vi "Set Combobox Items.vi"(6 "Combo Box Ref":refnum<vi>, 8 "error in (no error)":errorcluster, 9 "Run Mode?":bool, 10 "Indicator?":bool, 11 "Static Path Selector in":refnum<class "MGI Static Path Selector.lvclass">) -> (0 "error out":errorcluster, 2 "Strings And Values []":T1, 3 "Static Path Selector out":refnum<class "MGI Static Path Selector.lvclass">)   [LabVIEW 2020, in "MGI Static Path Selector.lvclass"]
doc: "Sets the Combobox strings to appropriate values for the specified state of the XControl.\n\nAuthored by Shawn Walpole\nsupport@mooregoodideas.com\nwww.mooregoodideas.com\n\nCopyright (c) 2013, Moore Good Ideas, Inc.\n\nAll rights reserved.\n\nRedistribution and use in source and binary forms, with or without modification, are permitted provided that the following conditions are met:\n\n * Redistributions of source code must retain the above copyright notice, this list of conditions and the following disclaimer.\n * Redistributions in binary form must reproduce the above copyright notice, this list of conditions and the following disclaimer in the documentation and/or other materials provided with the distribution.\n * Neither the name of Moore Good Ideas, Inc. nor the names of its contributors may be used to endorse or promote products derived from this software without specific prior written permission.\n\nTHIS SOFTWARE IS PROVIDED BY THE COPYRIGHT HOLDERS AND CONTRIBUTORS \"AS IS\" AND ANY EXPRESS OR IMPLIED WARRANTIES, INCLUDING, BUT NOT LIMITED TO, THE IMPLIED WARRANTIES OF MERCHANTABILITY AND FITNESS FOR A PARTICULAR PURPOSE ARE DISCLAIMED. IN NO EVENT SHALL THE COPYRIGHT OWNER OR CONTRIBUTORS BE LIABLE FOR ANY DIRECT, INDIRECT, INCIDENTAL, SPECIAL, EXEMPLARY, OR CONSEQUENTIAL DAMAGES (INCLUDING, BUT NOT LIMITED TO, PROCUREMENT OF SUBSTITUTE GOODS OR SERVICES; LOSS OF USE, DATA, OR PROFITS; OR BUSINESS INTERRUPTION) HOWEVER CAUSED AND ON ANY THEORY OF LIABILITY, WHETHER IN CONTRACT, STRICT LIABILITY, OR TORT (INCLUDING NEGLIGENCE OR OTHERWISE) ARISING IN ANY WAY OUT OF THE USE OF THIS SOFTWARE, EVEN IF ADVISED OF THE POSSIBILITY OF SUCH DAMAGE."
uses:
  <userlib>/_MGI/User Interface/Path Selector XControl/Class Hierarchy/Static File Selector/MGI Static Path Selector.lvclass
  <vilib>/Utility/miscctls.llb/LVComboBoxStrsAndValuesArrayTypeDef.ctl
  <userlib>/_MGI/User Interface/Path Selector XControl/Class Hierarchy/Static File Selector/MGI Static Path Selector.lvclass/MGI Static Path Selector.ctl
panel:
  in  "Configure":cluster{string, string}[](array[cluster])=[{"Configure...", "<Configure>"}]
  in  "Select, Explorer, Separator":cluster{string, string}[](array[cluster])=[{"Select...", "<Browse>"}, {"Explorer...", "<Explore>"}, {"-", "<->"}]
  # "These controls could be localized:"
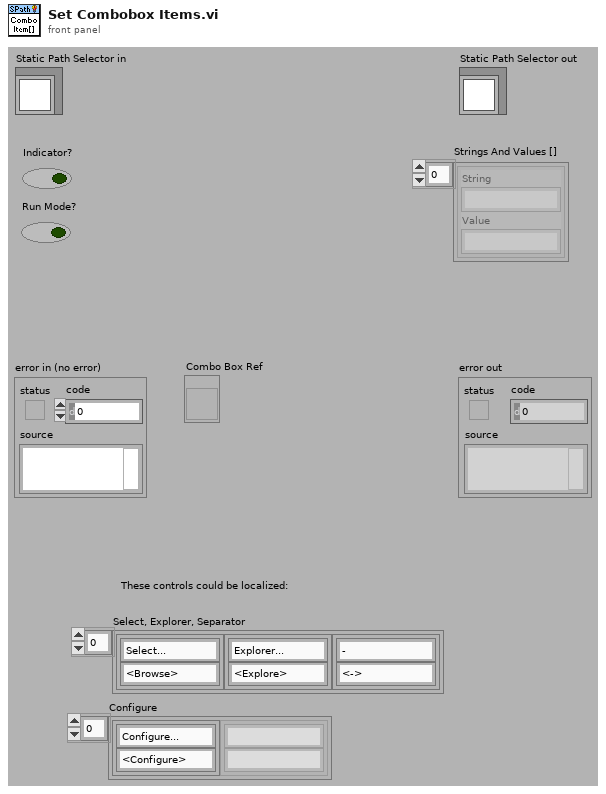
[diagram p1: front panel]
types:
  T1 = typedef "LVComboBoxStrsAndValuesArrayTypeDef.ctl" = cluster{"String":string, "Value":string}[]
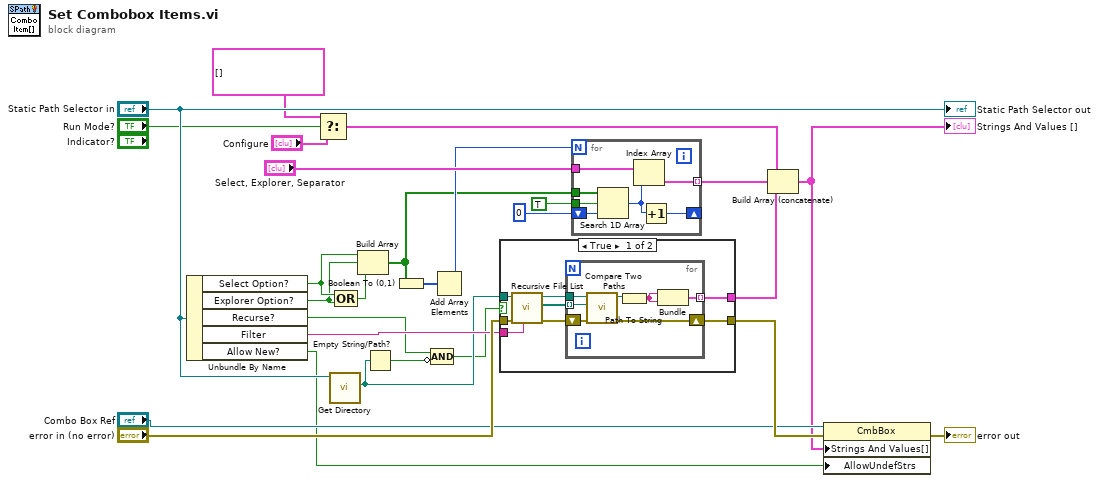
[diagram p0: block diagram]
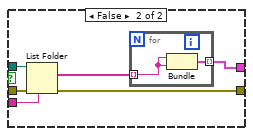
[diagram p2: hidden frame]
diagram:
  n1 = Unbundle By Name("Static Path Selector in") -> ("Select Option?"=w18:bool, "Explorer Option?"=w17:bool, "Recurse?"=w7:bool, "Filter"=w20:string, "Allow New?"=w1:bool)
  n2 = Select(t=cluster{string, string}[] [] ("element"), s="Run Mode?", f="Configure") -> (s? t:f=w3:cluster{string, string}[])
  n3 = call-dynamic "Get Directory.vi"("Static Path Selector"="Static Path Selector in") -> ("Start Path"=w9:path)  [unwired: 9 in, 1 out]
  n4 = Compound Arithmetic op=OR(w18, w17) -> (w16:bool)
  n5 = Build Array(w18, w17, w16) -> (w12:bool[])
  n6 = Empty String/Path?(string/path=w9) -> (empty?=w8:bool)
  n7 = Boolean To (0,1)(Boolean=w12) -> (0, 1=w15:i16[])
  n8 = Compound Arithmetic op=AND(w7, invert w8) -> (w6:bool)
  n9 = Add Array Elements(numeric array=w15) -> (sum=w14:i16)
  n10 = case shown="True" w6 {
    tunnel: w20 -> [w35 w46]
    tunnel: w9 -> [w34 w47]
    tunnel: "error in (no error)" -> [w33 w45]
    tunnel: [w29 w43] -> w24
    tunnel: [w28 w48] -> w19
    frame True {
      n11 = call <vilib>:"Recursive File List.vi"("pattern"=w35, "error in (no error)"=w33, "Folder Path"=w34) -> ("error out"=w30:errorcluster, "All Files in Dir"=w32:path[], "dup Folder Path"=w31:path)  [unwired: 4 in, 2 out]
      n12 = for {
        tunnel: w32 -> [w42] mode=indexing
        tunnel: w31 -> [w41]
        shift-right: [w39] -> w29
        shift-left: w30 -> [w40]
        tunnel: [w36] -> w28 mode=indexing
        n13 = call <vilib>:"Compare Two Paths.vi"("error in (no error)"=w40, "Path 2"=w42, "Path 1"=w41) -> ("error out"=w39:errorcluster, "Relative Path from 1 to 2"=w38:path)  [unwired: 5 in, 2 out]
        n14 = Path To String(path=w38) -> (string=w37:string)
        n15 = Bundle(w37, w37) -> (w36:cluster{string, string})  [unwired: 1 in]
      }
    }
    frame False {
      n16 = List Folder(path=w47, pattern=w46, error in=w45) -> (filenames=w44:string[], error out=w43:errorcluster)  [unwired: 1 in, 2 out]
      n17 = for {
        tunnel: [w50] -> w48 mode=indexing
        tunnel: w44 -> [w49] mode=indexing
        n18 = Bundle(w49, w49) -> (w50:cluster{string, string})  [unwired: 1 in]
      }
    }
  }
  n19 = for {
    N: w14 -> [_]
    shift-right: [w51] -> _
    shift-left: 0 -> [w56]
    tunnel: "Select, Explorer, Separator" -> [w54]
    tunnel: w12 -> [w57]
    tunnel: TRUE ("element") -> [w55]
    tunnel: [w53] -> w10 mode=indexing
    n20 = Search 1D Array(1D array=w57, element=w55, start index (0)=w56) -> (index of element=w52:i32)
    n21 = Index Array(array=w54, index=w52) -> (element=w53:cluster{string, string})
    n22 = Increment(x=w52) -> (x+1=w51:i32)
  }
  n23 = Build Array (concatenate)(w3, w10, w19) -> (w22:cluster{string, string}[])
  "Strings And Values []" <- w22
  n24 = property class="CmbBox"(reference="Combo Box Ref", error in=w24, "Strings And Values[]"=w22, "AllowUndefStrs"=w1) -> (error out=→"error out":errorcluster)  [unwired: 1 out]
  "Static Path Selector out" <- "Static Path Selector in"
